vi "Assert True.vi"(4 "Execution time (s)":dbl=-1.0, 6 "error code (1)":i32=1, 7 "Label":string, 8 "error in":errorcluster, 11 "True?":bool) -> (0 "error out":errorcluster, 2 "Properties":refnum<class "Properties.Assert.lvclass">)   [LabVIEW 2021, in "Bananas.lvlib"]
uses:
  Bananas.lvlib
  <vilib>/addons/_JKI Toolkits/Caraya/classes/Properties.Assert/Properties.Assert.lvclass
  Banana/Banana.lvclass/Banana.ctl
  AssertTrue/AssertTrue.lvclass
  C:/Repositories/LVOS/Bananas/lv-src/Bananas/BananaPeel/BananaPeel.lvclass
  <vilib>/addons/_JKI Toolkits/Caraya/classes/Assert/Assert.lvclass
  Banana/Banana.lvclass
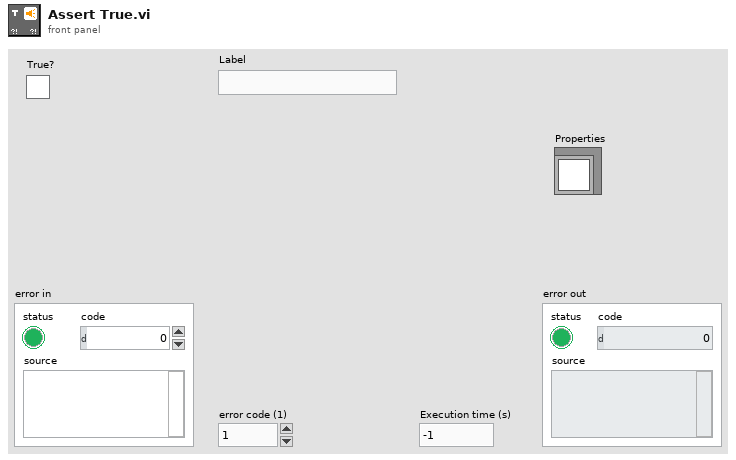
[diagram p1: front panel]
types:
  T1 = typedef "Bananas.lvlib/Assertion Strategies -- cluster.ctl" = cluster{"AssertTrue":refnum<class "AssertTrue.lvclass">, "AssertFalse":refnum<class "AssertFalse.lvclass">}
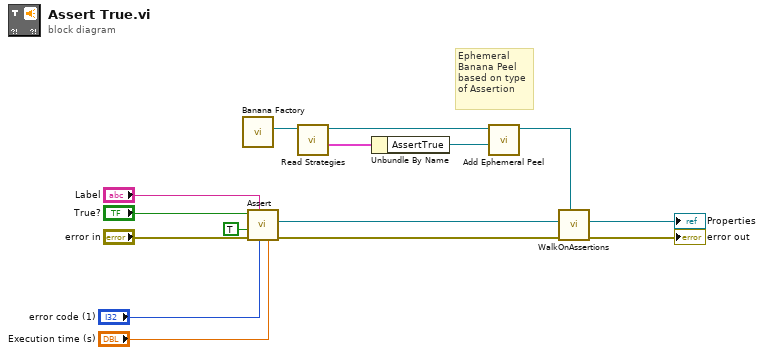
[diagram p0: block diagram]
diagram:
  # "Ephemeral\nBanana Peel\nbased on type\nof Assertion"
  n1 = call "Banana Factory.vi"() -> ("Bunch"=w3:refnum<class "Banana.lvclass">)  [unwired: 10 in, 1 out]
  n2 = call-poly <vilib>:"Assert.vi"("Execution time (s)"="Execution time (s)", "error code (1)"="error code (1)", "Label"="Label", "error in (no error)"="error in", "Register with caller test (F)"=TRUE, "True?"="True?") -> ("error out"=w9:errorcluster, "Properties"=w7:refnum<class "Properties.Assert.lvclass">)  [unwired: 4 in]
  n3 = call "Read Strategies.vi"("Banana in"=w3) -> ("Strategies"=w1:T1, "Banana out"=w2:refnum<class "Banana.lvclass">)  [unwired: 9 in]
  n4 = Unbundle By Name(w1) -> ("AssertTrue"=w4:refnum<class "AssertTrue.lvclass">)
  n5 = call "Add Ephemeral Peel.vi"("BananaPeel"=w4, "Bunch"=w2) -> ("Bunch"=w5:refnum<class "Banana.lvclass">)  [unwired: 9 in]
  n6 = call "WalkOnAssertions.vi"("Bunch"=w5, "error in (no error)"=w9, "Properties"=w7) -> ("error out"=→"error out":errorcluster, "Properties out"=→"Properties":refnum<class "Properties.Assert.lvclass">)  [unwired: 7 in]
